vi "Работа с CVS( exel) файлом knob вариант 2.vi"() -> ()   [LabVIEW 2021]
panel:
  out "output 4":i32
  out "output 3":i32
  out "output 2":string
  out "output 1":string
  in  "file path (dialog if empty)":path
  in  "Knob":dbl(knob) scale=0.0..10.0
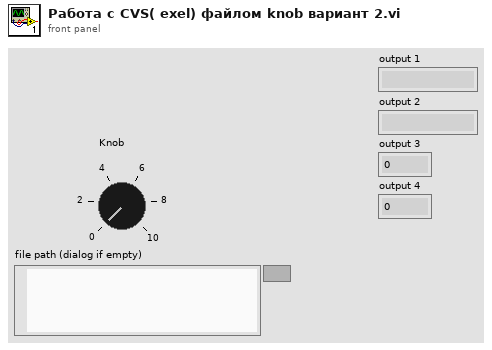
[diagram p1: front panel]
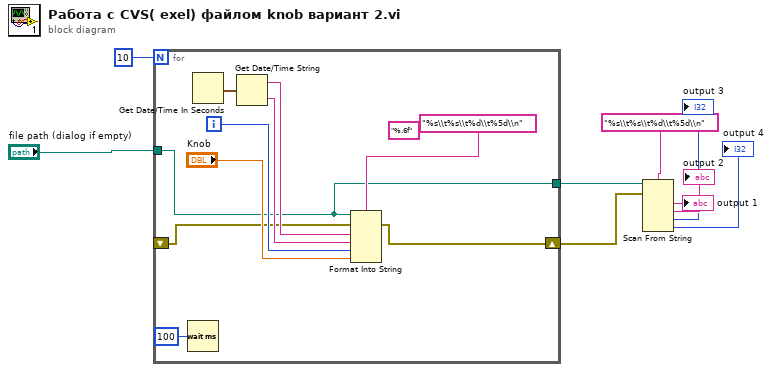
[diagram p0: block diagram]
diagram:
  n1 = for {
    N: 10 -> [_]
    shift-right: [w16] -> w2
    shift-left: _ -> [w11]
    tunnel: "file path (dialog if empty)" -> [w10]
    tunnel: [w10] -> w1
    i -> [w13]
    (unwired) "%.6f" ("format (%.3f)")
    n2 = Wait (ms)(milliseconds to wait=u32 100) -> ()  [unwired: 1 out]
    n3 = Get Date/Time In Seconds() -> (seconds since 1Jan1904=w18:timestamp)
    n4 = Get Date/Time String(seconds (now)=w18) -> (date string=w15:string, time string=w14:string)  [unwired: 2 in]
    n5 = Format Into String(format string="%s\\t%s\\t%d\\t%5d\\n", initial string=w10, error in=w11, w15, w14, w13, "Knob") -> (error out=w16:errorcluster)  [unwired: 1 out]
  }
  n6 = Scan From String("%s\\t%s\\t%d\\t%5d\\n" ("format string"), w1, w2) -> (output 1=→"output 1":string, output 2=→"output 2":string, output 3=→"output 3":i32, output 4=→"output 4":i32)  [unwired: 4 in, 2 out]
